vi "enumToStr.ProcHead.vi"(10 "Proc var":T1=enum."procIndex") -> (2 "String":string)   [LabVIEW 2024]
uses:
  controls/typeProcVarientName.ctl
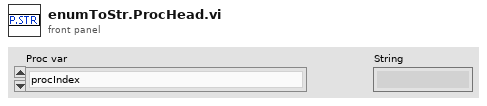
[diagram p1: front panel]
types:
  T1 = typedef "typeProcVarientName.ctl" = enum16{"procNameID", "procModuleID", "procPath", "procIsRunning", "procIndex", "procModule", "procRegisterNumeric", "procRegisterString", "procReport", "procReportPrev", "procCLK", "procStepPointer", "procType"}
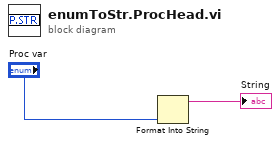
[diagram p0: block diagram]
diagram:
  n1 = Format Into String("Proc var") -> (resulting string=→"String":string)  [unwired: 3 in, 1 out]
